vi "write_attributes.vi"(8 "error in (no error)":errorcluster caption="entrée d'erreur (pas d'erreur)", 10 "attributes":T1, 11 "LinearRegression en entrée":refnum<class "LinearRegression.lvclass">) -> (0 "error out":errorcluster caption="sortie d'erreur", 3 "LinearRegression en sortie":refnum<class "LinearRegression.lvclass">)   [LabVIEW 2020, in "LinearRegression.lvclass"]
uses:
  LinearRegression.lvclass
  Controls/linear_regression_attributes.ctl
  LinearRegression.lvclass/LinearRegression.ctl
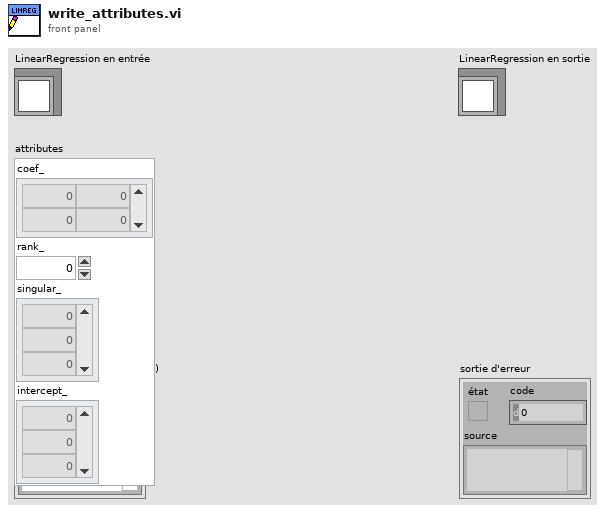
[diagram p1: front panel]
types:
  T1 = typedef "linear_regression_attributes.ctl" = cluster{"coef_":dbl[][], "rank_":dbl, "singular_":dbl[], "intercept_":dbl[]}
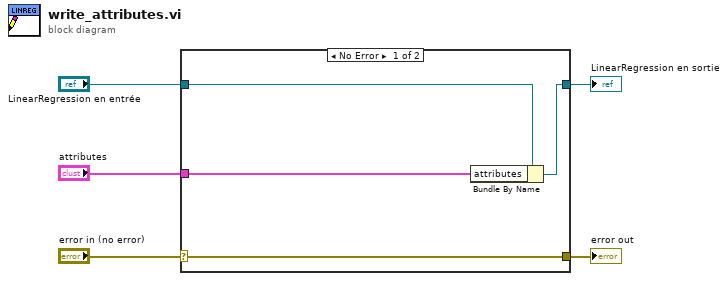
[diagram p0: block diagram]
diagram:
  n1 = case shown="No Error" "error in (no error)" {
    selector: "error in (no error)" -> [w9 w10]
    tunnel: [w9 w10] -> w4
    tunnel: [w7 w11] -> w2
    tunnel: "LinearRegression en entrée" -> [w8 w11]
    tunnel: "attributes" -> [w6 _]
    frame No Error {
      n2 = Bundle By Name(cluster=w8, "attributes"=w6) -> (w7:refnum<class "LinearRegression.lvclass">)
    }
    frame Error {
    }
  }
  "error out" <- w4
  "LinearRegression en sortie" <- w2
